vi "Is Active.vi"(10 "cycle count":u64=1, 11 "Transfer Group in":refnum<class "Transfer Group.lvclass">) -> (2 "active this cycle?":bool, 3 "Transfer Group out":refnum<class "Transfer Group.lvclass">)   [LabVIEW 2019, in "DSF Core.lvlib" / "Transfer Group.lvclass"]
uses:
  Transfer Group.lvclass
  Transfer Group.lvclass/Transfer Group.ctl
  Timing/Timing.lvclass
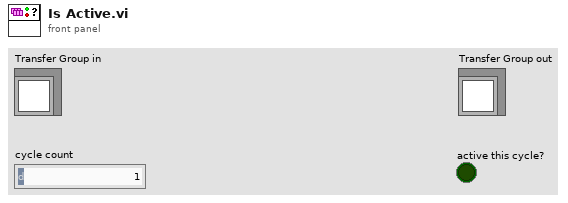
[diagram p1: front panel]
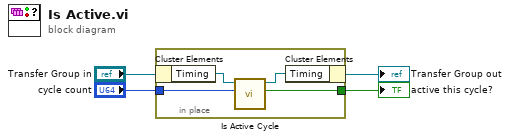
[diagram p0: block diagram]
diagram:
  n1 = in-place {
    in-place-border: "cycle count" -> [w8]
    in-place-border: [w7] -> w3
    n2 = in-place-cluster #1("Transfer Group in") -> ("Timing"=w6:refnum<class "Timing.lvclass">)
    n3 = call "Is Active Cycle.vi"("iteration"=w8, "Timing in"=w6) -> ("active?"=w7:bool, "Timing out"=w5:refnum<class "Timing.lvclass">)  [unwired: 8 in]
    n4 = in-place-cluster #1("Timing"=w5) -> (→"Transfer Group out":refnum<class "Transfer Group.lvclass">)
  }
  "active this cycle?" <- w3
